vi "read_OSC.vi"() -> ()   [LabVIEW 2011]
doc: "Demonstrates how to set up an oscilloscope automatically. You can configure this VI to acquire a waveform from a single channel by following the following steps:\n\n1. Specify a valid VISA resource to use. \n2. Specify a channel. \n3. Specify a time-out value for reading a waveform.\n4. Run this VI. The <B>Waveform Graph</B> displays the waveform you acquire."
uses:
  <instrlib>/Tektronix 7000 Series/Public/Data/Read (Single Waveform).vi
  <instrlib>/Tektronix 7000 Series/Tektronix 7000 Series.lvlib
panel:
  in  "Sampling Modes (Real Time)":u16(ring) items=["Real Time", "Interpolater", "Equivalent"]
  in  "Acquisition Type":u16(ring) items=["Sample", "Peak Detect", "Hi Res", "Average", "Envelope", "WfmDB"]
  in  "Average#":i32=10
  in  "Envelope Waveforms":i32=10
  in  "OSC":refnum<visa-resource-name>
  in  "Maximum Time":u32=10000
  in  "Meas Channel":u16(ring) items=["Channel 1", "Channel 2", "Channel 3", "Channel 4", "Math 1", "Math 2", "Math 3", "Math 4", "Reference 1", "Reference 2", "Reference 3", "Reference 4"]
  out "Waveform Graph":waveform(dbl)(graph)
  in  "STOP":bool
  in  "start":bool
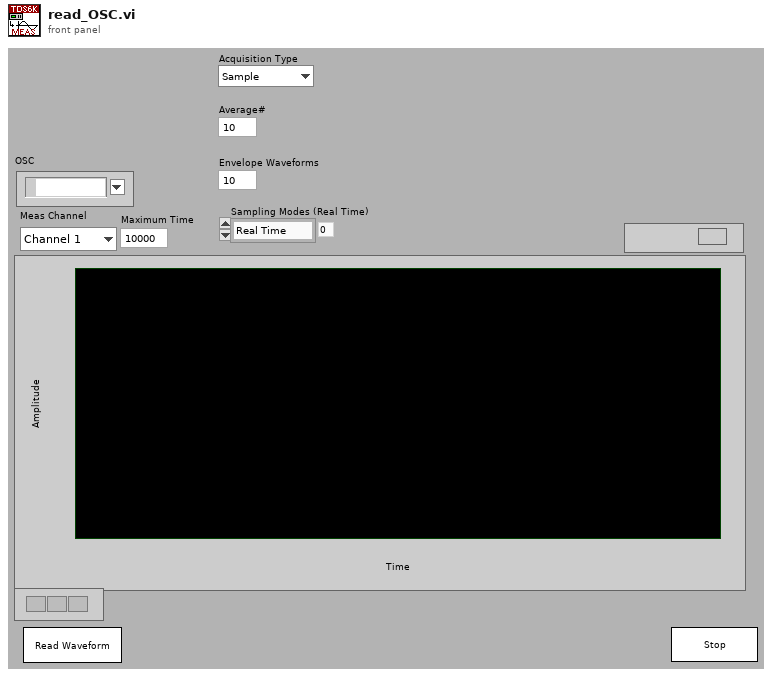
[diagram p1: front panel]
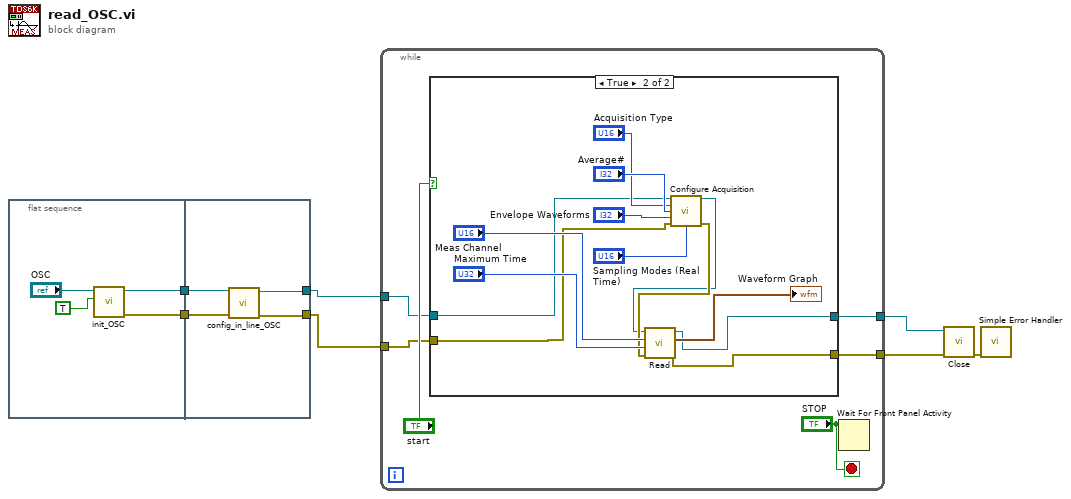
[diagram p0: block diagram]
diagram:
  n1 = flat-sequence {
    tunnel: [w9] -> w7
    tunnel: [w8] -> w6
    tunnel: [w13] -> w5
    tunnel: w7 -> [w15]
    tunnel: [w12] -> w4
    tunnel: w6 -> [w14]
    frame #0 {
      n2 = call "init_OSC.vi"("reset (f)"=TRUE, "VISA resource name"="OSC") -> ("error out"=w8:errorcluster, "VISA resource name out"=w9:refnum<visa-resource-name>)  [unwired: 8 in]
    }
    frame #1 {
      n3 = call "config_in_line_OSC.vi"("error in (no error)"=w14, "OSC 2"=w15) -> ("error out"=w12:errorcluster, "VISA resource name out"=w13:refnum<visa-resource-name>)  [unwired: 8 in]
    }
  }
  n4 = while {
    tunnel: w5 -> [w19]
    tunnel: w4 -> [w18]
    tunnel: [w17] -> w2
    tunnel: [w16] -> w1
    stop <- "STOP" stop-if-true
    n5 = case shown="True" "start" {
      tunnel: w19 -> [w23 w27]
      tunnel: w18 -> [w22 w26]
      tunnel: [w23 w25] -> w17
      tunnel: [w22 w24] -> w16
      frame False {
      }
      frame True {
        n6 = call <instrlib>:"Configure Acquisition.vi"("VISA resource name"=w27, "Acquisition Type (0:Sample)"="Acquisition Type", "Average Waveforms (10)"="Average#", "Envelope Waveforms (10)"="Envelope Waveforms", "error in (no error)"=w26, "Sampling Modes (Real Time)"="Sampling Modes (Real Time)") -> ("VISA resource name out"=w28:refnum<visa-resource-name>, "error out"=w29:errorcluster)  [unwired: 8 in]
        n7 = call-poly <instrlib>:"Read.vi"("error in (no error)"=w29, "Maximum Time (10000 ms)"="Maximum Time", "Channel (0: Channel 1)"="Meas Channel", "VISA resource name"=w28) -> ("error out"=w24:errorcluster, "Waveform Data"=→"Waveform Graph":waveform(dbl), "VISA resource name out"=w25:refnum<visa-resource-name>)  [unwired: 5 in]
      }
    }
    n8 = Wait For Front Panel Activity(3:"STOP") -> ()  [unwired: 2 in, 1 out]
  }
  n9 = call <instrlib>:"Close.vi"("error in (no error)"=w1, "VISA resource name"=w2) -> ("error out"=w3:errorcluster)  [unwired: 9 in]
  n10 = call <vilib>:"Simple Error Handler.vi"("error in (no error)"=w3) -> ()  [unwired: 4 in, 5 out]
